vi "segundo_programa.vi"() -> ()   [LabVIEW 2013]
panel:
  out "temperatura k":dbl
  out "temperatura f":dbl
  out "Thermometer 3":dbl(slide) scale=0.0..500.0
  out "Thermometer 2":dbl(slide) scale=0.0..100.0
  out "temperatura c":dbl
  in  "valor mv / c\nsensor temperatura":dbl
  out "Thermometer":dbl(slide) scale=0.0..100.0
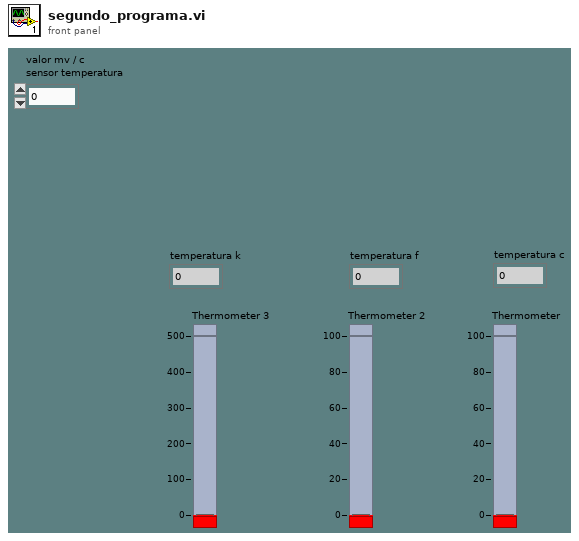
[diagram p1: front panel]
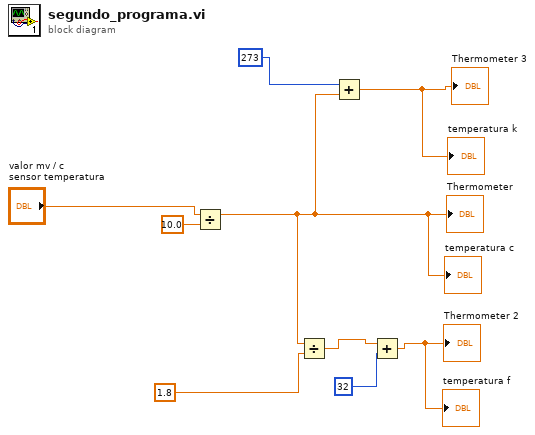
[diagram p0: block diagram]
diagram:
  n1 = Divide(x="valor mv / c\nsensor temperatura", y=10.0) -> (x/y=w6:dbl)
  "Thermometer" <- w6
  "temperatura c" <- w6
  n2 = Divide(x=w6, y=1.8) -> (x/y=w4:dbl)
  n3 = Add(x=273, y=w6) -> (x+y=→"Thermometer 3" →"temperatura k":dbl)
  n4 = Add(x=w4, y=32) -> (x+y=→"Thermometer 2" →"temperatura f":dbl)
